vi "Multi-Delete.vi"(1 "Element to Delete":dbl format="%#_13g", 2 "Input Array":dbl[](array[numeric])) -> (0 "Output Array":dbl[](array[numeric]))   [LabVIEW 2017]
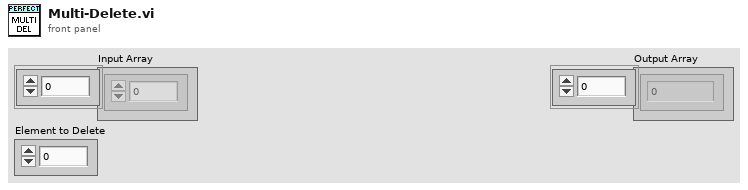
[diagram p1: front panel]
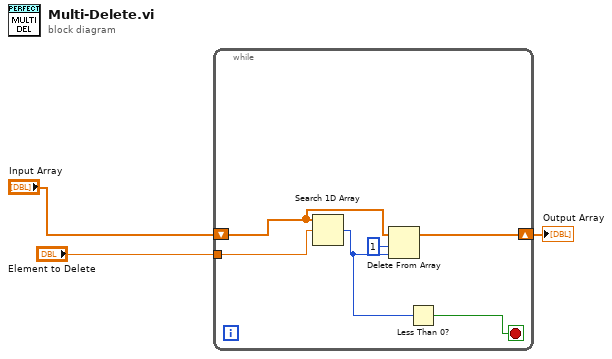
[diagram p0: block diagram]
diagram:
  n1 = while {
    tunnel: "Element to Delete" -> [w5]
    shift-right: [w4] -> w1
    shift-left: "Input Array" -> [w9]
    stop <- w6 stop-if-true
    n2 = Search 1D Array(1D array=w9, element=w5) -> (index of element=w7:i32)  [unwired: 1 in]
    n3 = Delete From Array(array=w9, length=1, index=w7) -> (array with subset deleted=w4:dbl[])  [unwired: 1 out]
    n4 = Less Than 0?(x=w7) -> (x < 0?=w6:bool)
  }
  "Output Array" <- w1
